vi "SetupSerialOpen.vi"(7 "Access Mode":T1=1 items=["VISA Defaults"=0, "Exclusive Lock"=1, "Load Configured Settings"=4], 8 "error in (no error)":errorcluster, 9 "flow control (0:none)":u16(ring) items=["None", "XON/XOFF", "RTS/CTS", "XON/XOFF & RTS/CTS", "DTR/DSR", "XON/XOFF & DTR/DSR"], 10 "Baud":dbl=115200.0, 11 "VISA Refnum in":refnum<visa-resource-name>) -> (0 "error out":errorcluster, 3 "VISA session":refnum<visa-resource-name>)   [LabVIEW 2013]
uses:
  <vilib>/Instr/_visa.llb/VISA Open Access Mode.ctl
  <vilib>/Instr/_visa.llb/VISA Configure Serial Port (Instr).vi
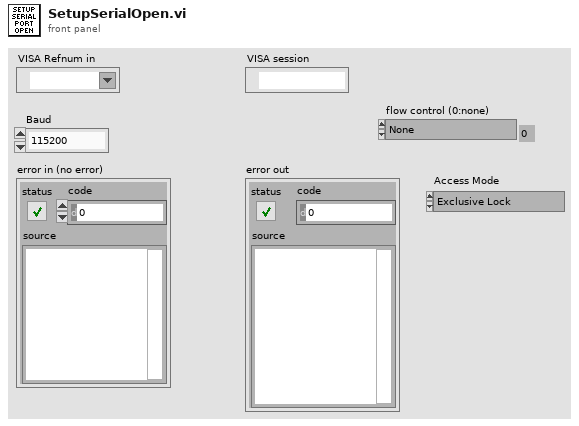
[diagram p1: front panel]
types:
  T1 = typedef "VISA Open Access Mode.ctl" = u32
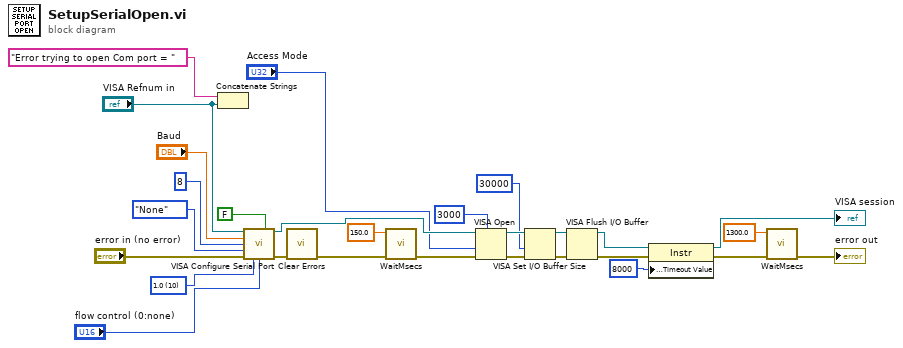
[diagram p0: block diagram]
diagram:
  w28 = u16 10 items=["1.0"=10, "1.5"=15, "2.0"=20] ("stop bits (10: 1 bit)")
  n1 = Concatenate Strings("Error trying to open Com port = " ("string"), "VISA Refnum in") -> ()  [unwired: 1 out]
  n2 = call-poly "VISA Configure Serial Port"("VISA resource name"="VISA Refnum in", "Enable Termination\nChar (T)"=FALSE ("Enable Termination\nChar (T)"), "baud rate (9600)"="Baud", "data bits (8)"=u16 8, "parity (0:none)"=enum16{"None", "Odd", "Even", "Mark", "Space"}."None", "error in (no error)"="error in (no error)", "stop bits (10: 1 bit)"=w28, "flow control (0:none)"="flow control (0:none)") -> ("VISA resource name out"=w24:refnum<visa-resource-name>, "error out"=w17:errorcluster)  [unwired: 6 in]
  n3 = call <vilib>:"Clear Errors.vi"("error in (no error)"=w17) -> ("error out"=w16:errorcluster)  [unwired: 6 in]
  n4 = call "WaitMsecs.vi"("error in (no error)"=w16, "Wait Msecs"=150.0) -> ("error out"=w7:errorcluster)  [unwired: 9 in]
  n5 = VISA Open(timeout (0)=u32 3000 ("VISA Open timeout (0)"), access mode="Access Mode", error in (no error)=w7, VISA resource name=w24) -> (VISA resource name=w5:refnum<visa-resource-name>, error out=w4:errorcluster)  [unwired: 1 in]
  n6 = VISA Set I/O Buffer Size(VISA resource name=w5, size (4096)=u32 30000, error in (no error)=w4) -> (VISA resource name out=w1:refnum<visa-resource-name>, error out=w2:errorcluster)  [unwired: 1 in]
  n7 = VISA Flush I/O Buffer(VISA resource name=w1, error in (no error)=w2) -> (VISA resource name out=w6:refnum<visa-resource-name>, error out=w11:errorcluster)  [unwired: 1 in]
  n8 = property class="Instr"(reference=w6, error in=w11, "General Settings:Timeout Value"=u32 8000) -> (reference out=→"VISA session":refnum<visa-resource-name>, error out=w12:errorcluster)
  n9 = call "WaitMsecs.vi"("error in (no error)"=w12, "Wait Msecs"=1300.0) -> ("error out"=→"error out":errorcluster)  [unwired: 9 in]
